vi "Label Name From Number And SDI.vi"(9 "SDI value":u8, 10 "label (Dec)":u32) -> (2 "label name":string)   [LabVIEW 2024, in "ARINC 429 Import.lvlib"]
uses:
  ARINC 429 Import.lvlib
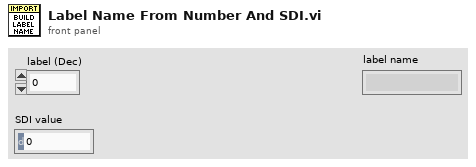
[diagram p1: front panel]
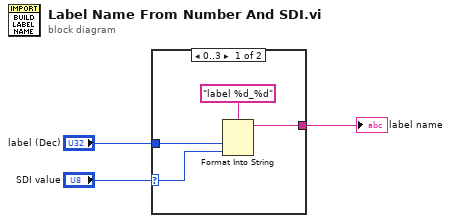
[diagram p0: block diagram]
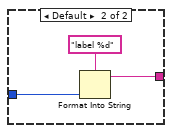
[diagram p2: hidden frame]
diagram:
  n1 = case shown="0..3" "SDI value" {
    selector: "SDI value" -> [w7 _]
    tunnel: "label (Dec)" -> [w5 w9]
    tunnel: [w4 w8] -> w2
    frame 0..3 {
      n2 = Format Into String(format string="label %d_%d", w5, w7) -> (resulting string=w4:string)  [unwired: 2 in, 1 out]
    }
    frame Default {
      n3 = Format Into String(format string="label %d", w9) -> (resulting string=w8:string)  [unwired: 2 in, 1 out]
    }
  }
  "label name" <- w2
